vi "Create 3DRect.vi"(8 "error in (no error)":errorcluster, 9 "Color":u32(colorbox), 10 "Size":cluster{"Width":i32, "Height":i32}) -> (0 "error out":errorcluster, 3 "Rectangle3D out":refnum<class "Rectangle3D.lvclass">)   [LabVIEW 2016, in "Rectangle3D.lvclass"]
uses:
  Rectangle3D.lvclass
  C:/Program Files (x86)/National Instruments/LabVIEW 2016/vi.lib/LIEF/Forms/Shape/Shape.lvclass
  C:/Program Files (x86)/National Instruments/LabVIEW 2016/vi.lib/LIEF/Forms/Rectangle/Rectangle.lvclass
  C:/Program Files (x86)/National Instruments/LabVIEW 2016/vi.lib/LIEF/Forms/Layered Shape/Layered Shape.lvclass
  <vilib>/LIEF/Forms/Rectangle/Rectangle.lvclass
  <vilib>/LIEF/Forms/Shape/Shape.lvclass/Shape.ctl
  <vilib>/LIEF/Forms/Rectangle/Rectangle.lvclass/Rectangle.ctl
  <vilib>/LIEF/Forms/Layered Shape/Layered Shape.lvclass/Layered Shape.ctl
  Rectangle3D.lvclass/Rectangle3D.ctl
  <vilib>/LIEF/Forms/Shape/Write Color.vi
  <vilib>/LIEF/Forms/Rectangle/Write Filled.vi
  <vilib>/LIEF/Forms/Shape/Read Bounds.vi
  <vilib>/LIEF/Forms/Layered Shape/Write Overlays.vi
  <vilib>/LIEF/Forms/Shape/Shape.lvclass
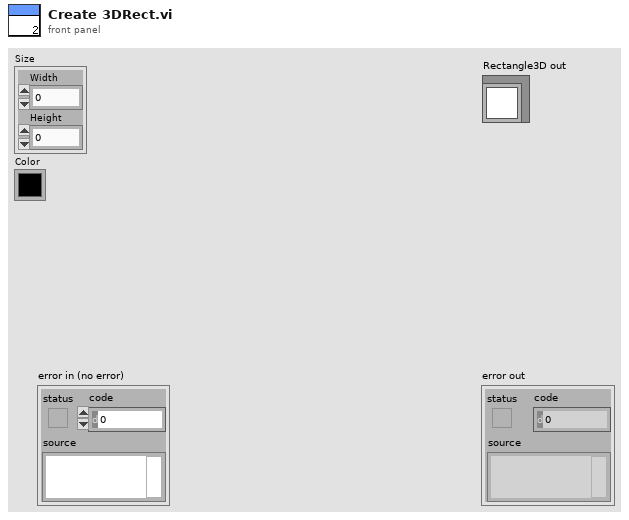
[diagram p1: front panel]
types:
  T1 = cluster{"Left":i32, "Top":i32, "Right":i32, "Bottom":i32}
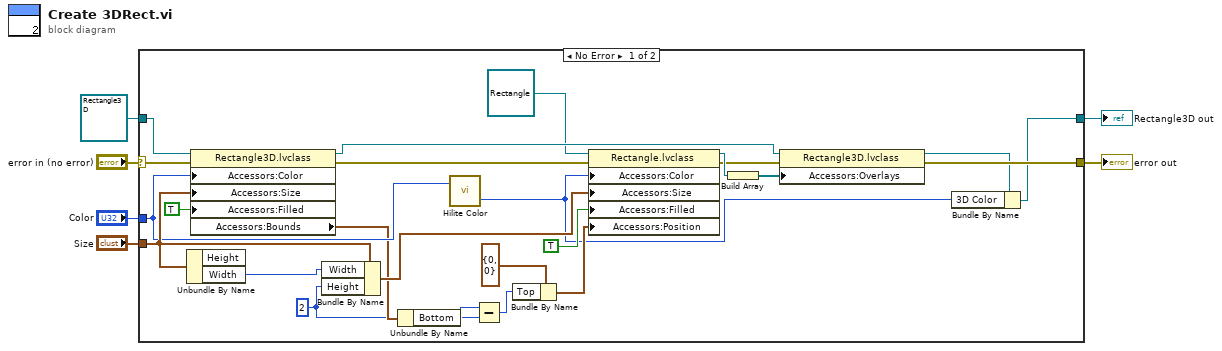
[diagram p0: block diagram]
diagram:
  n1 = case shown="No Error" "error in (no error)" {
    selector: "error in (no error)" -> [w20 w32]
    tunnel: [w17 w32] -> w5
    tunnel: [w8 w31] -> w1
    tunnel: refnum<class "Rectangle3D.lvclass"> refnum ("Rectangle3D out") -> [w24 w31]
    tunnel: "Size" -> [w19 _]
    tunnel: "Color" -> [w18 _]
    frame No Error {
      w12 = 2 ("Height")
      n2 = Unbundle By Name(w19) -> ("Width"=w30:i32)  [unwired: 1 out]
      n3 = property class="Rectangle3D.lvclass"(reference=w24, error in=w20, "Accessors:Color"=w18, "Accessors:Size"=w19, "Accessors:Filled"=TRUE ("Filled")) -> (reference out=w28:refnum<class "Rectangle3D.lvclass">, error out=w22:errorcluster, "Accessors:Bounds"=w15:T1)
      n4 = Bundle By Name(cluster=w19, "Width"=w30, "Height"=w12) -> (w29:cluster{"Width":i32, "Height":i32})
      n5 = Unbundle By Name(w15) -> ("Bottom"=w13:i32)
      n6 = call <vilib>:"Hilite Color.vi"("Color In"=w18) -> ("Shadow"=w7:u32)  [unwired: 1 in, 1 out]
      n7 = Subtract(x=w13, y=w12) -> (x-y=w11:i32)
      n8 = Bundle By Name(cluster=cluster{"Left":i32, "Top":i32} {"Left"=0, "Top"=0} ("Position"), "Top"=w11) -> (w10:cluster{"Left":i32, "Top":i32})
      n9 = property class="Rectangle.lvclass"(reference=refnum<class "Rectangle.lvclass"> refnum, error in=w22, "Accessors:Color"=w7, "Accessors:Size"=w29, "Accessors:Filled"=TRUE ("Filled"), "Accessors:Position"=w10) -> (reference out=w27:refnum<class "Rectangle.lvclass">, error out=w21:errorcluster)
      n10 = Build Array(w27) -> (w26:refnum<class "Rectangle.lvclass">[])
      n11 = property class="Rectangle3D.lvclass"(reference=w28, error in=w21, "Accessors:Overlays"=w26) -> (reference out=w9:refnum<class "Rectangle3D.lvclass">, error out=w17:errorcluster)
      n12 = Bundle By Name(cluster=w9, "3D Color"=w7) -> (w8:refnum<class "Rectangle3D.lvclass">)
    }
    frame Error {
    }
  }
  "error out" <- w5
  "Rectangle3D out" <- w1
